vi "Check for Calibration Values.vi"(8 "error in (no error)":errorcluster, 11 "File Name":string) -> (0 "error out":errorcluster, 2 "Intercept out":dbl, 3 "Slope out":dbl)   [LabVIEW 2020, in "SubVIs.lvlib"]
uses:
  SubVIs.lvlib
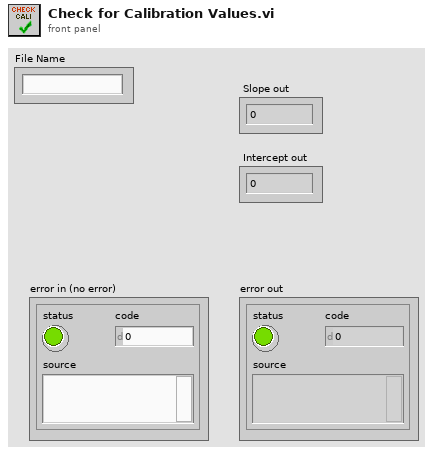
[diagram p1: front panel]
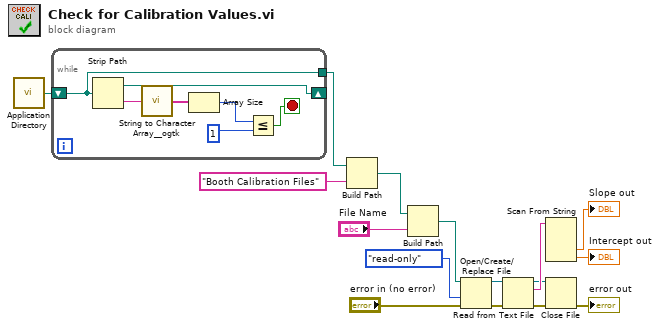
[diagram p0: block diagram]
diagram:
  n1 = call <vilib>:"Application Directory.vi"() -> ("Application Directory"=w6:path)
  n2 = while {
    shift-right: [w22] -> _
    shift-left: w6 -> [w23]
    tunnel: [w23] -> w4
    stop <- w19 stop-if-true
    n3 = Strip Path(path=w23) -> (stripped path=w22:path, name=w20:string)
    n4 = call <userlib>:"String to Character Array__ogtk.vi"("Input String"=w20) -> ("Character Array"=w21:string[])
    n5 = Array Size(array=w21) -> (size(s)=w17:i32)
    n6 = Less Or Equal?(x=w17, y=1) -> (x <= y?=w19:bool)
  }
  n7 = Build Path(base path=w4, name or relative path="Booth Calibration Files") -> (appended path=w3:path)
  n8 = Build Path(base path=w3, name or relative path="File Name") -> (appended path=w1:path)
  n9 = Open/Create/Replace File(file path (use dialog)=w1, error in="error in (no error)", access (0:read/write)=enum16{"read/write", "read-only", "write-only"}."read-only") -> (refnum out=w9:refnum<file>, error out=w11:errorcluster)  [unwired: 3 in, 1 out]
  n10 = Read from Text File(file (use dialog)=w9, error in=w11) -> (refnum out=w8:refnum<file>, text=w10:string, error out=w12:errorcluster)  [unwired: 2 in, 1 out]
  n11 = Scan From String(input string=w10) -> (output 1=→"Slope out":dbl, output 2=→"Intercept out":dbl)  [unwired: 5 in, 3 out]
  n12 = Close File(refnum=w8, error in=w12) -> (error out=→"error out":errorcluster)  [unwired: 1 out]
